vi "VI Server_Get ControlsValue_ArrayInput_StringFormat.vi"(6 "Options":T1, 7 "Labels.Array":string[](array[string]), 8 "error in (no error)":errorcluster, 11 "VI Server Cluster":T2) -> (0 "error out":errorcluster, 1 "Values.Array.STR":string[](array[string]), 2 "Labels.Array.DUP":string[](array[string]), 3 "VI Server Cluster.DUP":T2, 5 "Bad label":string)   [LabVIEW 2020, in "VI Server Toolkit LV2013.lvlib"]
doc: "<B>VI Server_GetControlValues(ArrayInput_StringFormat.vi</B> converts data type of the selected GUI objects into string format. Arrays are converted into comma delimited string."
uses:
  VI Server Toolkit LV2013.lvlib
  VI Server_TypeDefs/VI Server_RefsCluster.ctl
  VI Server Libraries/VI Server Controls.llb/VI Server_GetSet Controls From String Format_Options.ctl
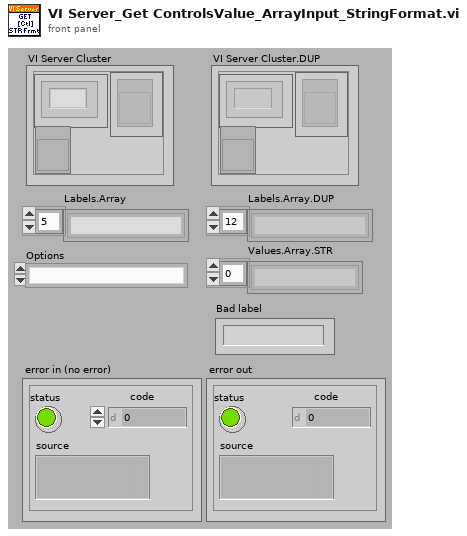
[diagram p1: front panel]
types:
  T1 = typedef "VI Server Toolkit LV2013.lvlib/VI Server_GetSet Controls From String Format_Options.ctl" = enum16{"", "If Ring Get Selection", "If Ring Set by Selection"}
  T2 = typedef "VI Server_RefsCluster.ctl" = cluster{"Labels":string[], "Refs":refnum<vi>[], "VI Ref":refnum<vi>}
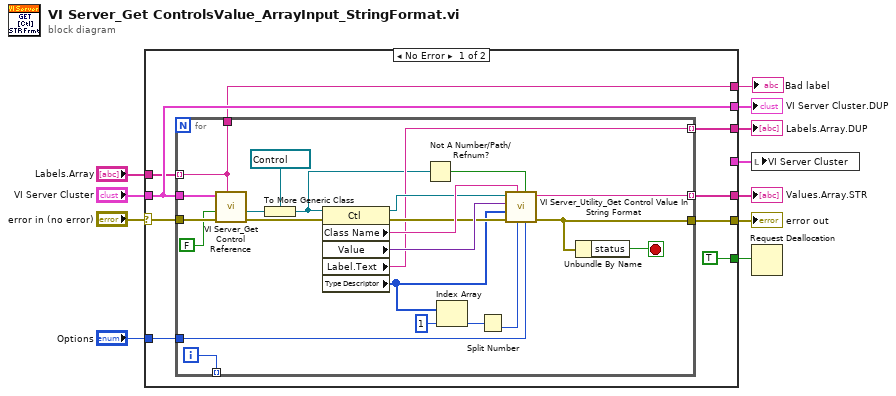
[diagram p0: block diagram]
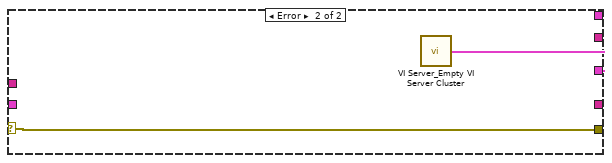
[diagram p2: hidden frame]
diagram:
  n1 = case shown="No Error" "error in (no error)" {
    selector: "error in (no error)" -> [w18 w45]
    tunnel: [w19 w45] -> w11
    tunnel: "VI Server Cluster" -> [w17 _]
    tunnel: "Labels.Array" -> [w16 _]
    tunnel: [w20 _] -> w7
    tunnel: [w17 _] -> w8
    tunnel: [w15 _] -> w5
    tunnel: "Options" -> [w14 _]
    tunnel: [TRUE _] -> w3
    tunnel: [_ w44] -> w2
    tunnel: [w12 _] -> w1
    frame No Error {
      n2 = for {
        tunnel: [w29] -> w20 mode=indexing
        tunnel: w17 -> [w35]
        tunnel: w16 -> [w24] mode=indexing
        tunnel: [w31] -> w15 mode=indexing
        tunnel: w14 -> [w30]
        tunnel: w18 -> [w37]
        tunnel: [w33] -> w19
        tunnel: [w24] -> w12
        tunnel: [w23] -> _ mode=indexing
        i -> [w23]
        stop <- w32 stop-if-true
        n3 = call "VI Server_Get Control Reference.vi"("Label"=w24, "error in"=w37, "Single Instance (T)"=FALSE, "VI Server Cluster"=w35) -> ("error out"=w36:errorcluster, "Control Reference (Generic)"=w21:refnum<vi>)  [unwired: 4 in, 2 out]
        n4 = To More Generic Class(target class=refnum<vi> refnum ("Control Reference (Generic)"), reference=w21) -> (generic class reference=w22:refnum<vi>)
        n5 = property class="Ctl"(reference=w22, error in=w36) -> (reference out=w39:refnum<vi>, error out=w38:errorcluster, "Class Name"=w43:string, "Value"=w42:variant, "Label.Text"=w31:string, "Type Descriptor"=w26:i16[])
        n6 = Not A Number/Path/Refnum?(number/path/refnum=w22) -> (NaN/Path/Refnum?=w34:bool)
        n7 = Index Array(array=w26, index=1) -> (element=w40:i16)
        n8 = Split Number(x=w40) -> (lo(x)=w27:u8)  [unwired: 1 out]
        n9 = call "VI Server_Utility_Get Control Value In String Format.vi"("Options"=w30, "Continue"=w34, "Control.Representation"=w27, "Control.ClassName"=w43, "error in (no error)"=w38, "TypeDesc"=w26, "Control.Value.Invariant"=w42, "Control.Ref"=w39) -> ("error out"=w33:errorcluster, "Control.String.OUT"=w29:string)  [unwired: 2 out]
        n10 = Unbundle By Name(w33) -> ("status"=w32:bool)
      }
    }
    frame Error {
      n11 = call "VI Server_Empty VI Server Cluster.vi"() -> ("VI Server Cluster"=w44:T2)  [unwired: 7 in]
    }
  }
  "error out" <- w11
  "VI Server Cluster.DUP" <- w8
  "Values.Array.STR" <- w7
  "Labels.Array.DUP" <- w5
  "Bad label" <- w1
  n12 = local write "VI Server Cluster"(w2) -> ()
  n13 = Request Deallocation(w3) -> ()
